vi "Write Time parameter.vi"(8 "error in (no error)":errorcluster, 10 "Time parameter":T1, 11 "Speed Mode in":refnum<class "Speed Mode.lvclass">) -> (0 "error out":errorcluster, 3 "Speed Mode out":refnum<class "Speed Mode.lvclass">)   [LabVIEW 2020, in "Speed Mode.lvclass"]
uses:
  Speed Mode.lvclass
  Speed Mode.lvclass/Speed Mode.ctl
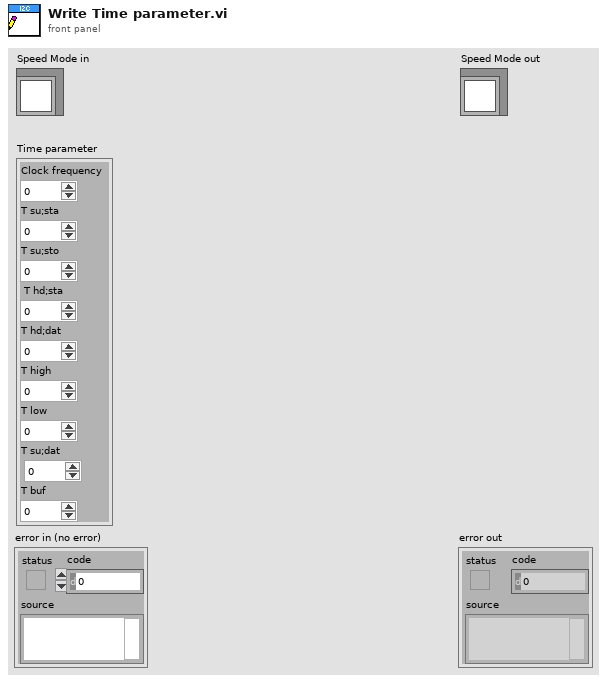
[diagram p1: front panel]
types:
  T1 = cluster{"Clock frequency":dbl, "T su;sta":dbl, "T su;sto":dbl, " T hd;sta":dbl, "T hd;dat":dbl, "T high":dbl, "T low":dbl, "T su;dat":dbl, "T buf":dbl}
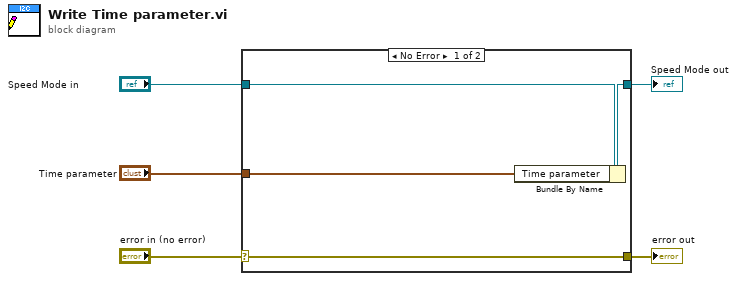
[diagram p0: block diagram]
diagram:
  n1 = case shown="No Error" "error in (no error)" {
    selector: "error in (no error)" -> [w9 w10]
    tunnel: [w9 w10] -> w4
    tunnel: [w7 w11] -> w2
    tunnel: "Speed Mode in" -> [w8 w11]
    tunnel: "Time parameter" -> [w6 _]
    frame No Error {
      n2 = Bundle By Name(cluster=w8, "Time parameter"=w6) -> (w7:refnum<class "Speed Mode.lvclass">)
    }
    frame Error {
    }
  }
  "error out" <- w4
  "Speed Mode out" <- w2
